vi "Watflow F4 System Setup.vi"() -> ()   [LabVIEW 2010]
doc: "This VI sets the system parameters which define the global operating characteristics of the controller.\n\nNote: It represents the <B>Main>Setup>System</B> menu of the controller."
uses:
  SubVIs/Watflow F4/Watflow F4.lvlib
panel:
  in  "Power-Out Action (0: Continue)":u16(ring) items=["Continue", "Hold", "Terminate", "Reset", "Idle Set Point 1", "Idle Set Point 2"]
  in  "Power-Out Time (10.0)":dbl=10.0 format="%.2f"
  in  "Open Loop Channel (F: Off)":bool
  in  "Input Fail (0.0)":dbl format="%.2f"
  in  "Channel Autotune Set Point (90.0)":dbl=90.0 format="%.2f"
  in  "Show °C or °F (T: Yes)":bool=TRUE
  in  "Temperature Scale (0: °F)":u16(ring) items=["°F", "°C"]
  in  "PID Units (0: US)":u16(ring) items=["US", "SI"]
  in  "Guarantee Soak Band (1.0)":dbl=1.0 format="%.2f"
  in  "Channel (1)":i16=1
  in  "Unit Address (1)":u8=1
  in  "Instrument Resource Name":refnum<visa-resource-name>
  in  "error in (no error)":errorcluster
  # "© 2005 National Instruments.  ALL RIGHTS RESERVED."
  # "WATLOW F4 Series"
  # "Main > Setup > System Parameters"
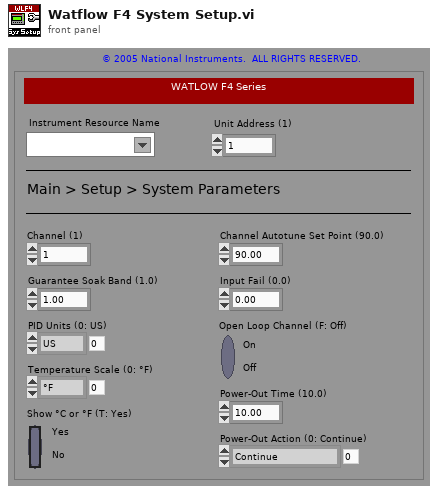
[diagram p1: front panel]
types:
  T1 = cluster{"second":i32, "minute":i32, "hour":i32, "day of month":i32, "month":i32, "year":i32, "day of week":i32, "day of year":i32, "is DST":i32}
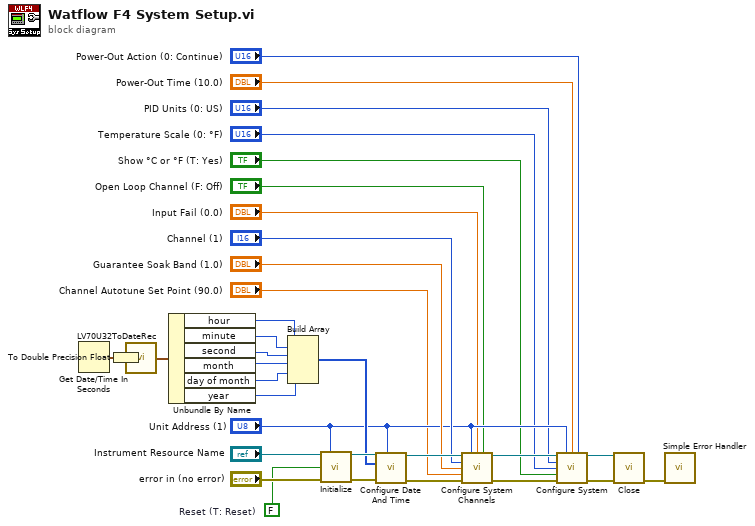
[diagram p0: block diagram]
diagram:
  w19 = FALSE  # Reset (T: Reset)
  n1 = Get Date/Time In Seconds() -> (seconds since 1Jan1904=w1:timestamp)
  n2 = To Double Precision Float(number=w1) -> (double precision float=w28:dbl)
  n3 = call <vilib>:"LV70U32ToDateRec.vi"("Time"=w28) -> ("date time rec"=w27:T1)
  n4 = Unbundle By Name(w27) -> ("hour"=w21:i32, "minute"=w22:i32, "second"=w23:i32, "month"=w24:i32, "day of month"=w25:i32, "year"=w26:i32)
  n5 = Build Array(w21, w22, w23, w24, w25, w26) -> (w20:i32[])
  n6 = call "Initialize.vi"("VISA resource name"="Instrument Resource Name", "Unit Address (1)"="Unit Address (1)", "Reset (T: Reset)"=w19, "error in (no error)"="error in (no error)") -> ("VISA resource name out"=w29:refnum<visa-resource-name>, "error out"=w30:errorcluster)  [unwired: 10 in]
  n7 = call "Configure Date And Time.vi"("Unit Address (1)"="Unit Address (1)", "error in (no error)"=w30, "Input Array (0; 0; 0; 1; 1; 2004)"=w20, "VISA resource name"=w29) -> ("error out"=w18:errorcluster, "VISA resource name out"=w17:refnum<visa-resource-name>)  [unwired: 6 in]
  n8 = call "Configure System Channels.vi"("VISA resource name"=w17, "Unit Address (1)"="Unit Address (1)", "Input Fail (0.0)"="Input Fail (0.0)", "Open Loop Channel (F: Off)"="Open Loop Channel (F: Off)", "Channel (1)"="Channel (1)", "Guarantee Soak Band (1.0)"="Guarantee Soak Band (1.0)", "Channel Autotune Set Point (90.0)"="Channel Autotune Set Point (90.0)", "error in (no error)"=w18) -> ("VISA resource name out"=w11:refnum<visa-resource-name>, "error out"=w14:errorcluster)  [unwired: 6 in]
  n9 = call "Configure System.vi"("VISA resource name"=w11, "Unit Address (1)"="Unit Address (1)", "Power-Out Time (10.0)"="Power-Out Time (10.0)", "Power-Out Action (0: Continue)"="Power-Out Action (0: Continue)", "PID Units (0: US)"="PID Units (0: US)", "Temperature Scale (0: °F)"="Temperature Scale (0: °F)", "Show °C or °F (T: Yes)"="Show °C or °F (T: Yes)", "error in (no error)"=w14) -> ("VISA resource name out"=w10:refnum<visa-resource-name>, "error out"=w13:errorcluster)  [unwired: 6 in]
  n10 = call "Close.vi"("VISA resource name"=w10, "error in (no error)"=w13) -> ("error out"=w31:errorcluster)  [unwired: 13 in]
  n11 = call <vilib>:"Simple Error Handler.vi"("error in (no error)"=w31) -> ()  [unwired: 4 in, 5 out]
